vi "Build Data.vi"(8 "error in (no error)":errorcluster, 10 "Data":variant, 11 "Command":string) -> (0 "error out":errorcluster, 3 "UDP MSG To be Sent":string)   [LabVIEW 2021, in "UDP Comms.lvlib"]
uses:
  UDP Comms.lvlib
  UDP Message--cluster.ctl
  183e2ca8-03a9-4ddc-a228-d48b97ba419b.vi
  <vilib>/LabVIEW Open Source Project/Data Manipulation/TypeDescriptor/TypeDescriptor_SetName.vi
  <vilib>/JDP Science/JSONtext/Variant to JSON Text.vi
  <vilib>/JDP Science/JSONtext/LVClass Serializer/JSONtext LVClass Serializer.lvclass
  <vilib>/LabVIEW Open Source Project/Data Manipulation/Variant/OpenVariant.lvlib
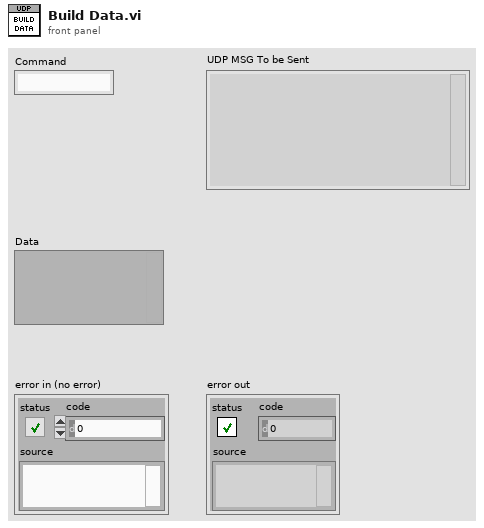
[diagram p1: front panel]
types:
  T1 = typedef "UDP Comms.lvlib/UDP Message--cluster.ctl" = cluster{"Command":string, "Data":variant}
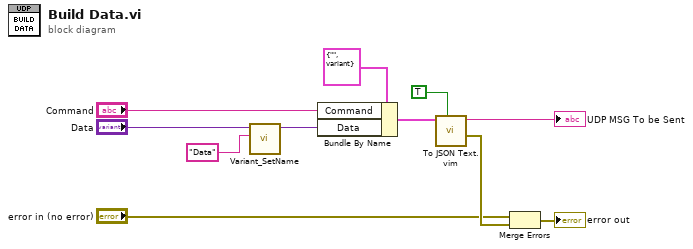
[diagram p0: block diagram]
diagram:
  n1 = call <vilib>:"Variant_SetName.vi"("Name"="Data", "Variant"="Data") -> ("Named Variant"=w5:variant)  [unwired: 9 in]
  n2 = Bundle By Name(cluster=T1 {"Command"="", "Data"=variant} ("Cluster"), "Command"="Command", "Data"=w5) -> (w11:T1)
  n3 = call "To JSON Text.vim"("enable LabVIEW extensions? (T)"=TRUE, "Anything"=w11) -> ("error out"=w3:errorcluster, "<JSON>"=→"UDP MSG To be Sent":string)  [unwired: 8 in]
  n4 = Merge Errors("error in (no error)", w3) -> (→"error out":errorcluster)
